vi "Wavegen set frequency.vi"(8 "error in (no error)":errorcluster, 9 "Frequency (Hz)":dbl=0.1 caption="Frequency" min=0.1, 11 "IVI Refnum in":refnum<k15>) -> (0 "error out":errorcluster, 2 "log string out":string, 3 "IVI Refnum out":refnum<k15>)   [LabVIEW 2021]
uses:
  <instrlib>/Keysight InfiniiVision/Keysight InfiniiVision.lvlib
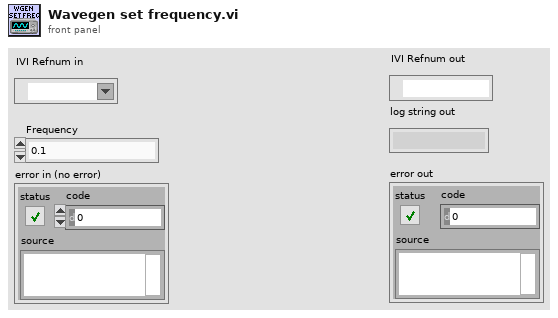
[diagram p1: front panel]
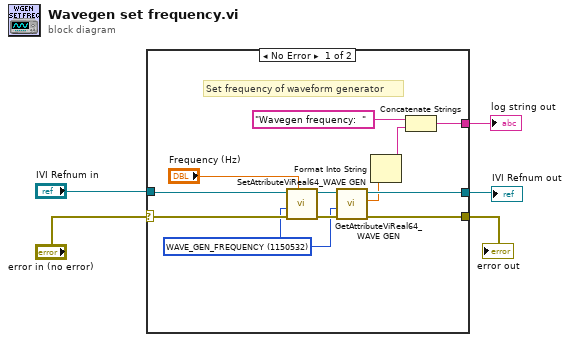
[diagram p0: block diagram]
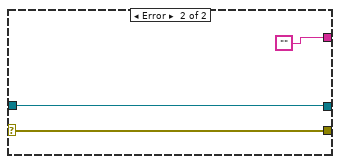
[diagram p2: hidden frame]
diagram:
  n1 = case shown="No Error" "error in (no error)" {
    selector: "error in (no error)" -> [w16 w19]
    tunnel: "IVI Refnum in" -> [w17 w20]
    tunnel: [w12 w19] -> w4
    tunnel: [w11 w20] -> w3
    tunnel: [w9 ""] -> w1
    frame No Error {
      w13 = u32 1150532 items=["FM_DEVIATION"=1150548, "FM_FREQUENCY"=1150549, "FSK_FREQUENCY"=1150550, "FSK_MODULATION_RATE"=1150551, "MODULATION_RAMP_SYMMETRY"=1150553, "WAVE_GEN_AM_DEPTH"=1150546, "WAVE_GEN_AM_FREQUENCY"=1150547, "WAVE_GEN_AMPLITUDE"=1150530, "WAVE_GEN_DUTY_CYCLE"=1150531, "WAVE_GEN_FREQUENCY"=1150532, "WAVE_GEN_HIGH_VOLTAGE"=1150534, "WAVE_GEN_LOW_VOLTAGE"=1150535, "WAVE_GEN_OFFSET_VOLTAGE"=1150536, "WAVE_GEN_PERIOD"=1150539, "WAVE_GEN_PULSE_WIDTH"=1150540, "WAVE_GEN_RAMP_SYMMETRY"=1150541] ("AttributeID")
      # "Set frequency of waveform generator"
      n2 = call <instrlib>:"SetAttributeViReal64_WAVE GEN.vi"("AttributeValue"="Frequency (Hz)", "error in (no error)"=w16, "AttributeID"=w13, "instrument handle"=w17) -> ("error out"=w14:errorcluster, "instrument handle out"=w15:refnum<k15>)  [unwired: 6 in]
      n3 = call <instrlib>:"GetAttributeViReal64_WAVE GEN.vi"("error in (no error)"=w14, "AttributeID"=w13, "instrument handle"=w15) -> ("error out"=w12:errorcluster, "AttributeValue"=w7:dbl, "instrument handle out"=w11:refnum<k15>)  [unwired: 6 in]
      n4 = Format Into String(w7) -> (resulting string=w6:string)  [unwired: 3 in, 1 out]
      n5 = Concatenate Strings("Wavegen frequency:  ", w6) -> (w9:string)
    }
    frame Error {
    }
  }
  "error out" <- w4
  "IVI Refnum out" <- w3
  "log string out" <- w1
